vi "Quadratic Programming IP.vi"(4 "stopping criteria":T1={"function tolerance"=1e-08, "parameter tolerance"=1000000.0, "max iterations"=10000, "max function calls"=10000, "gradient tolerance"=1000000.0, "max time (sec)"=-1.0}, 6 "inequality constraints":cluster{"D":dbl[][], "Imin":dbl[], "Imax":dbl[]}, 7 "start":dbl[](array[numeric]), 8 "error in (no error)":errorcluster, 9 "equality constraints":cluster{"A":dbl[][], "b":dbl[]}, 10 "parameter bounds":cluster{"Xmin":dbl[], "Xmax":dbl[]}, 11 "objective function":cluster{"Q":dbl[][], "c":dbl[]}) -> (0 "error out":errorcluster, 1 "lagrangian multipliers":dbl[](array[numeric]), 2 "f(minimum)":dbl, 3 "minimum":dbl[](array[numeric]))   [LabVIEW 2017, in "NI_Gmath.lvlib"]
doc: "Uses either an interior point algorithm or an active set algorithm to solve the problem: minimize 0.5x*Q*x + c*x, such that A*x=b and <B>Imin</B> are less than or equal to D*x, which is less than or equal to <B>Imax</B>. You must manually select the polymorphic instance to use."
uses:
  NI_Gmath.lvlib
  stopping criteria.ctl
  qp_problem data.ctl
  A x Vector.vi
  Real A x B.vi
  Matrix left divisionMV.vi
  Matrix left divisionMM.vi
  NI_AALBase.lvlib
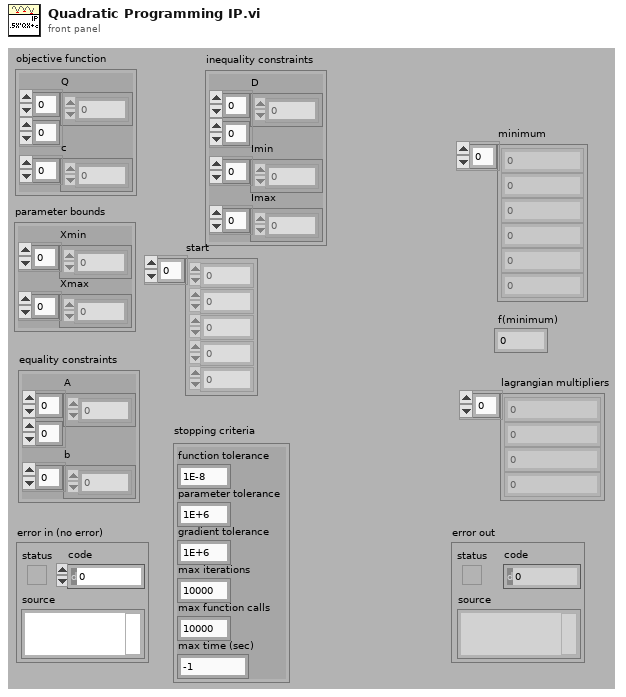
[diagram p1: front panel]
types:
  T1 = typedef "NI_Gmath.lvlib/stopping criteria.ctl" = cluster{"function tolerance":dbl, "parameter tolerance":dbl, "max iterations":i32, "max function calls":i32, "gradient tolerance":dbl, "max time (sec)":dbl}
  T2 = typedef "NI_Gmath.lvlib/qp_problem data.ctl" = cluster{"Q":dbl[][], "c":dbl[], "A":dbl[][], "b":dbl[], "Xmin":dbl[], "Xmax":dbl[], "M":i32, "N":i32, "D":dbl[][], "Imax":dbl[], "Imin":dbl[], "NI":i32, "X":dbl[]}
  T3 = typedef "NI_Gmath.lvlib/stopping criteria with time.ctl" = cluster{"function tolerance":dbl, "parameter tolerance":dbl, "max iterations":i32, "max function calls":i32, "gradient tolerance":dbl, "max time (sec)":dbl, "initial tick count":u32}
  T4 = typedef "NI_Matrix.lvlib/RealMatrix.ctl" = dbl[][]
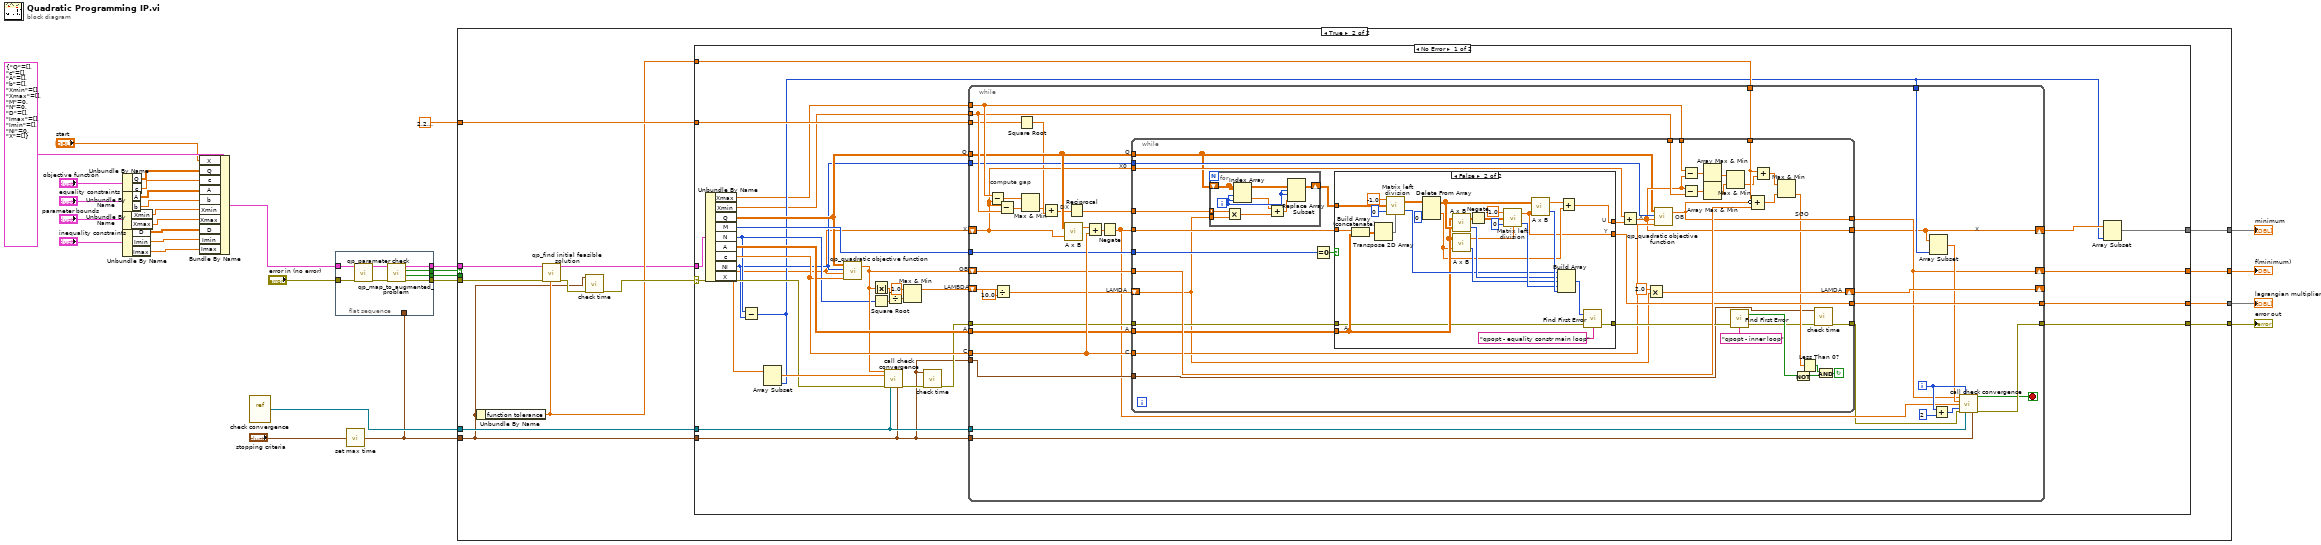
[diagram p0: block diagram]
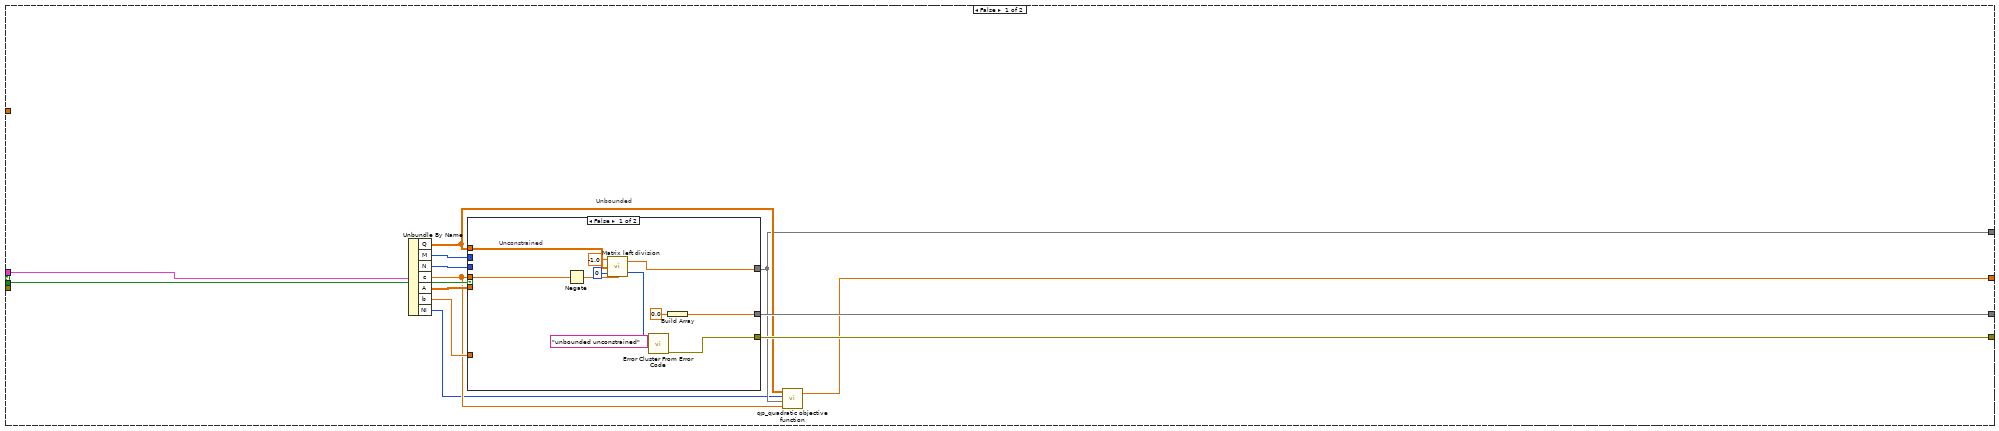
[diagram p2: hidden frame]
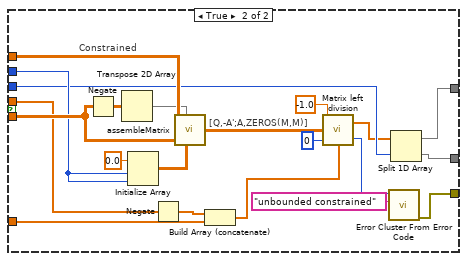
[diagram p3: hidden frame]
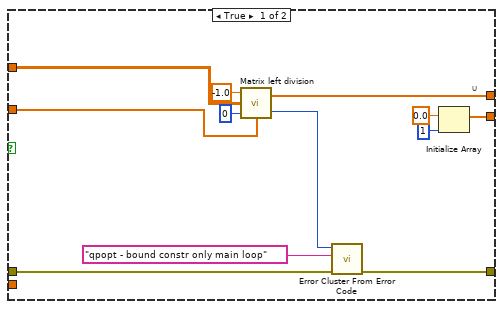
[diagram p4: hidden frame]
diagram:
  n1 = Unbundle By Name("parameter bounds") -> ("Xmin"=w20:dbl[], "Xmax"=w19:dbl[])
  n2 = Unbundle By Name("objective function") -> ("Q"=w24:dbl[][], "c"=w23:dbl[])
  n3 = Unbundle By Name("equality constraints") -> ("A"=w22:dbl[][], "b"=w21:dbl[])
  n4 = Unbundle By Name("inequality constraints") -> ("D"=w18:dbl[][], "Imin"=w17:dbl[], "Imax"=w16:dbl[])
  n5 = Bundle By Name(cluster=T2 {"Q"=[], "c"=[], "A"=[], "b"=[], "Xmin"=[], "Xmax"=[], "M"=0, "N"=0, "D"=[], "Imax"=[], "Imin"=[], "NI"=0, "X"=[]} ("qp data"), "X"="start", "Q"=w24, "c"=w23, "A"=w22, "b"=w21, "Xmin"=w20, "Xmax"=w19, "D"=w18, "Imin"=w17, "Imax"=w16) -> (w8:T2)
  n6 = vi-ref "check convergence.vi"() -> ("vi reference"=w9:refnum<vi>)
  n7 = flat-sequence {
    tunnel: "error in (no error)" -> [w37]
    tunnel: w8 -> [w36]
    tunnel: [w35] -> w7
    tunnel: [w34] -> w6
    tunnel: [w33] -> w5
    tunnel: [w32] -> w4
    tunnel: w1 -> [_]
    frame #0 {
      n8 = call "qp_parameter check.vi"("error in (no error)"=w37, "qp data in"=w36) -> ("error out"=w31:errorcluster, "qp data in"=w30:T2)  [unwired: 8 in]
      n9 = call "qp_map_to_augmented_problem.vi"("error in (no error)"=w31, "qp data in"=w30) -> ("error out"=w35:errorcluster, "constrained?"=w33:bool, "bounded?"=w34:bool, "qp data out"=w32:T2)  [unwired: 6 in]
    }
  }
  n10 = call "set max time.vi"("stopping criteria"="stopping criteria") -> ("stopping criteria"=w1:T3)
  n11 = case shown="True" w6 {
    tunnel: w5 -> [w50 _]
    tunnel: [w41 w94] -> w26
    tunnel: [w49 w93] -> w29
    tunnel: [w39 w91] -> w28
    tunnel: 2.220446049250313e-16 -> [_ w95]
    tunnel: [w48 w92] -> w27
    tunnel: w4 -> [w43 w87]
    tunnel: w7 -> [_ w86]
    tunnel: w9 -> [_ w90]
    tunnel: w1 -> [_ w83]
    frame False {
      # "Unbounded"
      n12 = Unbundle By Name(w43) -> ("Q"=w42:dbl[][], "M"=w47:i32, "N"=w46:i32, "c"=w40:dbl[], "A"=w45:dbl[][], "b"=w44:dbl[], "NI"=w38:i32)
      n13 = case shown="False" w50 {
        tunnel: w40 -> [w61 w79]
        tunnel: w42 -> [w56 w82]
        tunnel: w45 -> [_ w81]
        tunnel: [w54 w76] -> w41
        tunnel: [w59 w75] -> w49
        tunnel: w47 -> [_ w80]
        tunnel: w44 -> [_ w78]
        tunnel: w46 -> [_ w77]
        tunnel: [w57 w74] -> w48
        frame False {
          # "Unconstrained"
          n14 = Negate(x=w61) -> (-x=w55:dbl[])
          n15 = call-poly "Matrix left division.vi"("A"=w55, "number of iterations"=0, "B"=w56, "SVD relative tolerance"=-1.0) -> ("error"=w53:i32, "B\\A"=w54:dbl[])
          n16 = call "Error Cluster From Error Code.vi"("error message (\"\")"="unbounded unconstrained" ("error message (\"\")"), "error code (0)"=w53) -> ("error out"=w57:errorcluster)  [unwired: 7 in]
          n17 = Build Array(0.0) -> (w59:dbl[])
        }
        frame True {
          # "[Q,-A';A,ZEROS(M,M)]"
          # "Constrained"
          n18 = Negate(x=w81) -> (-x=w73:dbl[][])
          n19 = Transpose 2D Array(2D array=w73) -> (transposed array=w70:dbl[][])
          n20 = Initialize Array(0.0 ("element"), w80, w80) -> (w69:dbl[][])
          n21 = Negate(x=w79) -> (-x=w71:dbl[])
          n22 = call "assembleMatrix.vi"("A"=w82, "B"=w70, "C"=w81, "D"=w69) -> ("ABCD"=w67:dbl[][])  [unwired: 1 in]
          n23 = Build Array (concatenate)(w71, w78) -> (w64:dbl[])
          n24 = call-poly "Matrix left division.vi"("A"=w64, "number of iterations"=0, "B"=w67, "SVD relative tolerance"=-1.0) -> ("error"=w65:i32, "B\\A"=w66:dbl[])
          n25 = call "Error Cluster From Error Code.vi"("error message (\"\")"="unbounded constrained" ("error message (\"\")"), "error code (0)"=w65) -> ("error out"=w74:errorcluster)  [unwired: 7 in]
          n26 = Split 1D Array(array=w66, index=w77) -> (first subarray=w76:dbl[], second subarray=w75:dbl[])
        }
      }
      n27 = call "qp_quadratic objective function.vi"("c"=w40, "X"=w41, "NI"=w38, "Q"=w42) -> ("ob"=w39:dbl)  [unwired: 1 in]
    }
    frame True {
      n28 = Unbundle By Name(w83) -> ("function tolerance"=w88:dbl)
      n29 = call "qp_find initial feasible solution.vi"("tolerance"=w88, "error in (no error)"=w86, "qp data in"=w87) -> ("error out"=w85:errorcluster, "qp data in"=w84:T2)  [unwired: 7 in]
      n30 = call "check time.vi"("error in (no error)"=w85, "stopping criteria"=w83) -> ("error out"=w89:errorcluster)  [unwired: 9 in]
      n31 = case shown="No Error" w89 {
        selector: w89 -> [w112 w252]
        tunnel: w95 -> [w122 _]
        tunnel: [w106 _] -> w94
        tunnel: [w121 _] -> w93
        tunnel: [w120 w252] -> w92
        tunnel: w84 -> [w105 _]
        tunnel: [w116 _] -> w91
        tunnel: w90 -> [w113 _]
        tunnel: w83 -> [w96 _]
        tunnel: w88 -> [w103 _]
        frame No Error {
          # "A"
          # "C"
          # "Q"
          # "X"
          # "OB"
          # "LAMBDA"
          n32 = Unbundle By Name(w105) -> ("Xmax"=w98:dbl[], "Xmin"=w99:dbl[], "Q"=w108:dbl[][], "M"=w119:i32, "N"=w102:i32, "A"=w118:dbl[][], "c"=w117:dbl[], "NI"=w101:i32, "X"=w97:dbl[])
          n33 = Subtract(x=w102, y=w101) -> (x-y=w100:i32)
          n34 = Array Subset(array=w97, length=w100) -> (w114:dbl[])  [unwired: 1 in]
          n35 = call "qp_quadratic objective function.vi"("c"=w117, "X"=w97, "NI"=w101, "Q"=w108) -> ("ob"=w115:dbl)  [unwired: 1 in]
          n36 = Absolute Value(x=w115) -> (abs(x)=w125:dbl)
          n37 = Square Root(x=w102) -> (sqrt(x)=w111:dbl)
          n38 = call "call check convergence.vi"("f"=w115, "X"=w114, "error in"=w112, "vi reference"=w113, "stopping criteria"=w96) -> ("error out"=w110:errorcluster)  [unwired: 6 in, 4 out]
          n39 = Divide(x=w125, y=w111) -> (x/y=w124:dbl)
          n40 = Max & Min(x=1.0, y=w124) -> (max(x,y)=w107:dbl)  [unwired: 1 out]
          n41 = call "check time.vi"("error in (no error)"=w110, "stopping criteria"=w96) -> ("error out"=w109:errorcluster)  [unwired: 9 in]
          n42 = while {
            shift-right: [w155] -> _
            shift-left: w107 -> [w160]
            shift-right: [w137] -> w116
            shift-left: w115 -> [w154]
            tunnel: w98 -> [w157]
            tunnel: w99 -> [w156]
            shift-right: [w128] -> w104
            shift-left: w97 -> [w149]
            tunnel: w122 -> [w135]
            tunnel: w108 -> [w151]
            tunnel: w117 -> [w164]
            tunnel: w119 -> [w161]
            tunnel: w118 -> [w158]
            tunnel: [w153] -> w121
            tunnel: [w142] -> w120
            tunnel: w109 -> [w152]
            tunnel: w101 -> [w148]
            tunnel: w100 -> [w146]
            tunnel: w113 -> [w141]
            tunnel: w96 -> [w140]
            tunnel: w96 -> [w136]
            tunnel: w103 -> [w131]
            i -> [w145]
            stop <- w139 stop-if-true
            # "Q"
            # "C"
            # "A"
            # "X"
            # "X0"
            # "LAMDA"
            # "DX"
            # "compute gap"
            n43 = Subtract(x=w157, y=w149) -> (x-y=w163:dbl[])
            n44 = Divide(x=w160, y=10.0) -> (x/y=w130:dbl)
            n45 = Subtract(x=w149, y=w156) -> (x-y=w162:dbl[])
            n46 = Square Root(x=w135) -> (sqrt(x)=w132:dbl)
            n47 = Max & Min(x=w163, y=w162) -> (min(x,y)=w129:dbl[])  [unwired: 1 out]
            n48 = Add(x=w129, y=w132) -> (x+y=w134:dbl[])
            n49 = call-poly "A x B.vi"("Vector"=w149, "A"=w151) -> ("A x Vector"=w150:dbl[])  [unwired: 1 out]
            n50 = Reciprocal(x=w134) -> (1/x=w133:dbl[])
            n51 = Add(x=w150, y=w164) -> (x+y=w147:dbl[])
            n52 = Negate(x=w147) -> (-x=w127:dbl[])
            n53 = while {
              tunnel: w151 -> [w175]
              tunnel: w161 -> [w202]
              shift-right: [w197] -> w155
              shift-left: w130 -> [w165]
              tunnel: w149 -> [w199]
              tunnel: w164 -> [w180]
              tunnel: w158 -> [w200]
              tunnel: w157 -> [w195]
              tunnel: w156 -> [w196]
              tunnel: w154 -> [w203]
              tunnel: w131 -> [w169]
              tunnel: [w176] -> w128
              tunnel: [w181] -> w137
              tunnel: [w188] -> w153
              tunnel: [w171] -> w126
              tunnel: w152 -> [w178]
              tunnel: w127 -> [w179]
              tunnel: w133 -> [w166]
              tunnel: w148 -> [w177]
              tunnel: w136 -> [w170]
              stop <- w182 continue-if-true
              # "X"
              # "LAMDA"
              # "SGO"
              # "OB"
              n54 = for {
                shift-right: [w206] -> w174
                shift-left: w175 -> [w211]
                tunnel: w165 -> [w205]
                tunnel: w166 -> [w209] mode=indexing
                i -> [w210]
                n55 = Multiply(x=w209, y=w205) -> (x*y=w208:dbl)
                n56 = Index Array(array=w211, index (row)=w210, index (col)=w210) -> (element=w204:dbl)
                n57 = Add(x=w204, y=w208) -> (x+y=w207:dbl)
                n58 = Replace Array Subset(array=w211, new element=w207, index (row)=w210, index (col)=w210) -> (w206:dbl[][])
              }
              n59 = Equal To 0?(x=w202) -> (x = 0?=w201:bool)
              n60 = case shown="False" w201 {
                tunnel: w174 -> [w217 w226]
                tunnel: w179 -> [w216 w241]
                tunnel: [w214 w243] -> w189
                tunnel: w200 -> [_ w240]
                tunnel: [w223 w233] -> w188
                tunnel: [w219 w236] -> w185
                tunnel: w178 -> [w218 w235]
                frame True {
                  # "U"
                  n61 = call-poly "Matrix left division.vi"("A"=w216, "number of iterations"=0, "B"=w217, "SVD relative tolerance"=-1.0) -> ("error"=w215:i32, "B\\A"=w214:dbl[])
                  n62 = call "Error Cluster From Error Code.vi"("error in (no error)"=w218, "error message (\"\")"="qpopt - bound constr only main loop" ("source messages"), "error code (0)"=w215) -> ("error out"=w219:errorcluster)  [unwired: 6 in]
                  n63 = Initialize Array(0.0 ("element"), 1 ("dimension size")) -> (w223:dbl[])
                }
                frame False {
                  # "A"
                  # "Y"
                  # "U"
                  n64 = Build Array (concatenate)(w241, w240) -> (w239:dbl[][])
                  n65 = Transpose 2D Array(2D array=w239) -> (transposed array=w227:dbl[][])
                  n66 = call-poly "Matrix left division.vi"("A"=w227, "number of iterations"=0, "B"=w226, "SVD relative tolerance"=-1.0) -> ("error"=w247:i32, "B\\A"=w228:dbl[][])
                  n67 = Delete From Array(array=w228, index (col)=0 ("disabled index (col)")) -> (deleted portion=w234:dbl[], array with subset deleted=w244:dbl[][])  [unwired: 2 in]
                  n68 = call-poly "A x B.vi"("B"=w244, "A"=w240) -> ("error"=w248:i32, "A x B"=w245:T4)
                  n69 = call-poly "A x B.vi"("Vector"=w234, "A"=w240) -> ("error"=w249:i32, "A x Vector"=w232:dbl[])
                  n70 = Negate(x=w245) -> (-x=w231:T4)
                  n71 = call-poly "Matrix left division.vi"("A"=w232, "number of iterations"=0, "B"=w231, "SVD relative tolerance"=-1.0) -> ("error"=w250:i32, "B\\A"=w233:dbl[])
                  n72 = call-poly "A x B.vi"("Vector"=w233, "A"=w244) -> ("error"=w251:i32, "A x Vector"=w242:dbl[])
                  n73 = Build Array(w247, w248, w249, w250, w251) -> (w237:i32[])
                  n74 = Add(x=w242, y=w234) -> (x+y=w243:dbl[])
                  n75 = call "Find First Error.vi"("error in (no error)"=w235, "source messages"="qpopt - equality constr main loop", "error codes"=w237) -> ("error out"=w236:errorcluster)  [unwired: 1 in, 1 out]
                }
              }
              n76 = Add(x=w199, y=w189) -> (x+y=w176:dbl[])
              n77 = Multiply(x=2.0, y=w165) -> (x*y=w197:dbl)
              n78 = call "qp_quadratic objective function.vi"("c"=w180, "X"=w176, "NI"=w177, "Q"=w175) -> ("ob"=w181:dbl)  [unwired: 1 in]
              n79 = Subtract(x=w195, y=w176) -> (x-y=w194:dbl[])
              n80 = Subtract(x=w176, y=w196) -> (x-y=w193:dbl[])
              n81 = Array Max & Min(array=w194) -> (min value=w192:dbl)  [unwired: 3 out]
              n82 = Array Max & Min(array=w193) -> (min value=w191:dbl)  [unwired: 3 out]
              n83 = Max & Min(x=w192, y=w191) -> (min(x,y)=w168:dbl)  [unwired: 1 out]
              n84 = call "Find First Error.vi"("error in (no error)"=w185, "source messages"="qpopt - inner loop") -> ("error out"=w172:errorcluster, "error?"=w184:bool)  [unwired: 2 in]
              n85 = Compound Arithmetic op=ADD(w169, invert w181, w203) -> (w190:dbl)
              n86 = Add(x=w169, y=w168) -> (x+y=w167:dbl)
              n87 = Max & Min(x=w167, y=w190) -> (min(x,y)=w173:dbl)  [unwired: 1 out]
              n88 = Not(x=w184) -> (.not. x?=w183:bool)
              n89 = Less Than 0?(x=w173) -> (x < 0?=w187:bool)
              n90 = call "check time.vi"("error in (no error)"=w172, "stopping criteria"=w170) -> ("error out"=w171:errorcluster)  [unwired: 9 in]
              n91 = And(x=w187, y=w183) -> (x .and. y?=w182:bool)
            }
            n92 = Array Subset(array=w128, length=w146) -> (w138:dbl[])  [unwired: 1 in]
            n93 = Add(x=w145, y=2) -> (x+y=w143:i32)
            n94 = call "call check convergence.vi"("f"=w137, "current iteration"=w145, "X"=w138, "gradient"=w127, "number of function evaluations"=w143, "error in"=w126, "vi reference"=w141, "stopping criteria"=w140) -> ("stop?"=w139:bool, "error out"=w142:errorcluster)  [unwired: 3 in, 3 out]
          }
          n95 = Array Subset(array=w104, length=w100) -> (w106:dbl[])  [unwired: 1 in]
        }
        frame Error {
        }
      }
    }
  }
  "minimum" <- w26
  "lagrangian multipliers" <- w29
  "f(minimum)" <- w28
  "error out" <- w27
